vi "MonitorForRunCount.vi"(8 "error in (no error)":errorcluster, 11 "Calculated Values":T1) -> (0 "error out":errorcluster)   [LabVIEW 2018, in "Controller (Host).lvlib"]
uses:
  Controller (Host).lvlib
  Top Level/Shared Controls/Calculated Data.ctl
  93de32e7-e00c-40e6-9e23-44152d43563b.vi
  File IO/File IO.lvlib
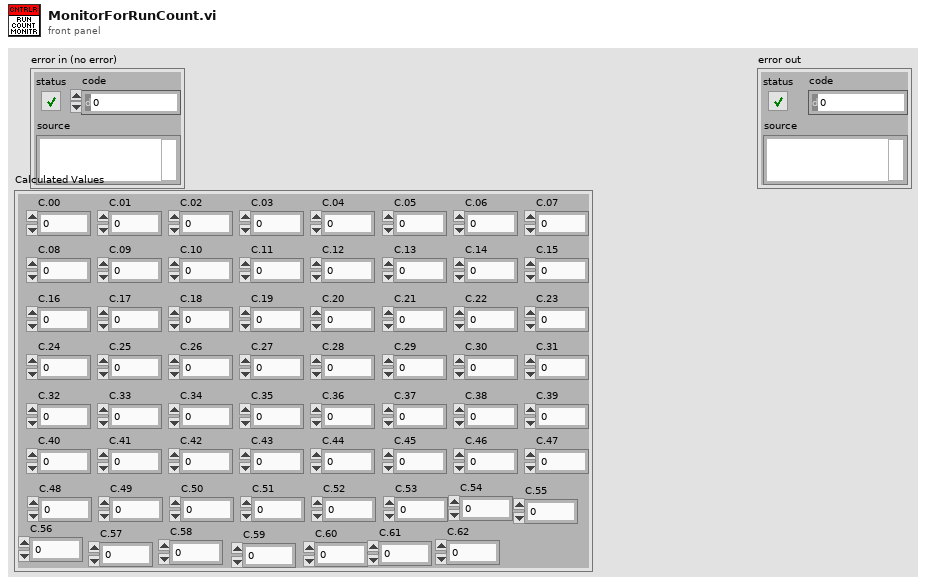
[diagram p1: front panel]
types:
  T1 = typedef "Calculated Data.ctl" = cluster{"C.00":dbl, "C.01":dbl, "C.02":dbl, "C.03":dbl, "C.04":dbl, "C.05":dbl, "C.06":dbl, "C.07":dbl, "C.08":dbl, "C.09":dbl, "C.10":dbl, "C.11":dbl, "C.12":dbl, "C.13":dbl, "C.14":dbl, "C.15":dbl, "C.16":dbl, "C.17":dbl, "C.18":dbl, "C.19":dbl, "C.20":dbl, "C.21":dbl, "C.22":dbl, "C.23":dbl, "C.24":dbl, "C.25":dbl, "C.26":dbl, "C.27":dbl, "C.28":dbl, "C.29":dbl, "C.30":dbl, "C.31":dbl, "C.32":dbl, "C.33":dbl, "C.34":dbl, "C.35":dbl, "C.36":dbl, "C.37":dbl, "C.38":dbl, "C.39":dbl, "C.40":dbl, "C.41":dbl, "C.42":dbl, "C.43":dbl, "C.44":dbl, "C.45":dbl, "C.46":dbl, "C.47":dbl, "C.48":dbl, "C.49":dbl, "C.50":dbl, "C.51":dbl, "C.52":dbl, "C.53":dbl, "C.54":dbl, "C.55":dbl, "C.56":dbl, "C.57":dbl, "C.58":dbl, "C.59":dbl, "C.60":dbl, "C.61":dbl, "C.62":dbl}
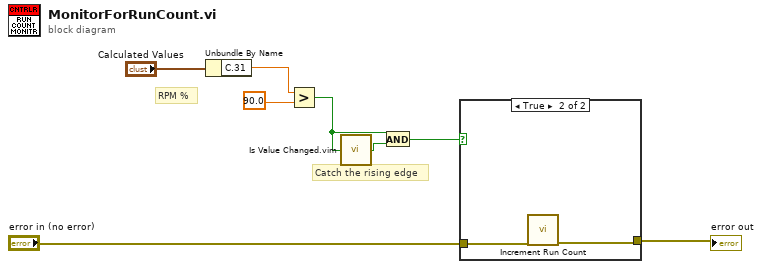
[diagram p0: block diagram]
diagram:
  # "Catch the rising edge"
  # "RPM %"
  n1 = Unbundle By Name("Calculated Values") -> ("C.31"=w4:dbl)
  n2 = Greater?(x=w4, y=90.0) -> (0:w2:bool)
  n3 = call "Is Value Changed.vim"("value"=w2) -> ("changed or first call?"=w1:bool)
  n4 = And(x=w2, y=w1) -> (x .and. y?=w6:bool)
  n5 = case shown="True" w6 {
    tunnel: "error in (no error)" -> [w9 w11]
    tunnel: [w9 w10] -> w8
    frame False {
    }
    frame True {
      n6 = call "Increment Run Count.vi"("error in (no error)"=w11) -> ("error out"=w10:errorcluster)  [unwired: 10 in]
    }
  }
  "error out" <- w8
